vi "Practica 7 Case 2_0.vi"() -> ()   [LabVIEW 2020]
panel:
  out "VENTILADOR":bool
  out "LED":bool
  out "FOCO":bool
  out "Temp":dbl
  out "Ring":u16(ring)
  out "MENSAJE DE ADVERTENCIA":string
  in  "Sensor":dbl(slide) scale=0.0..50.0
  in  "TEMP MAX":dbl
  in  "TEMP MIN":dbl
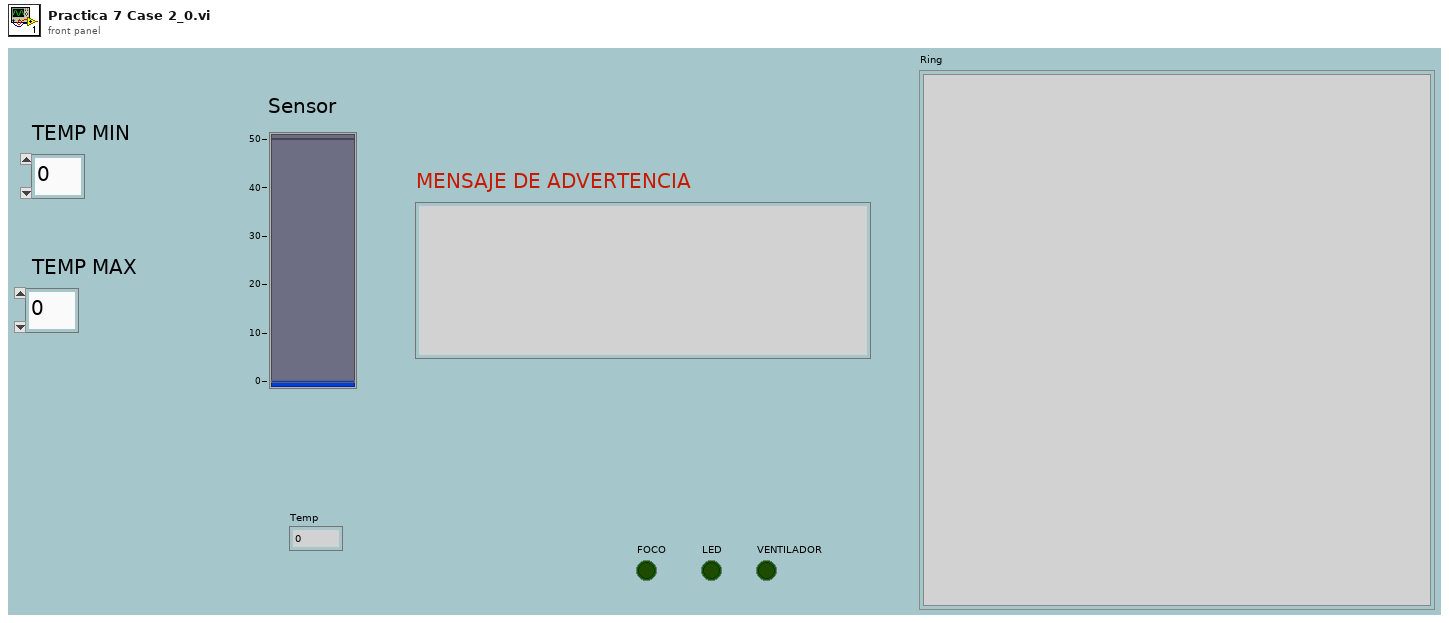
[diagram p1: front panel]
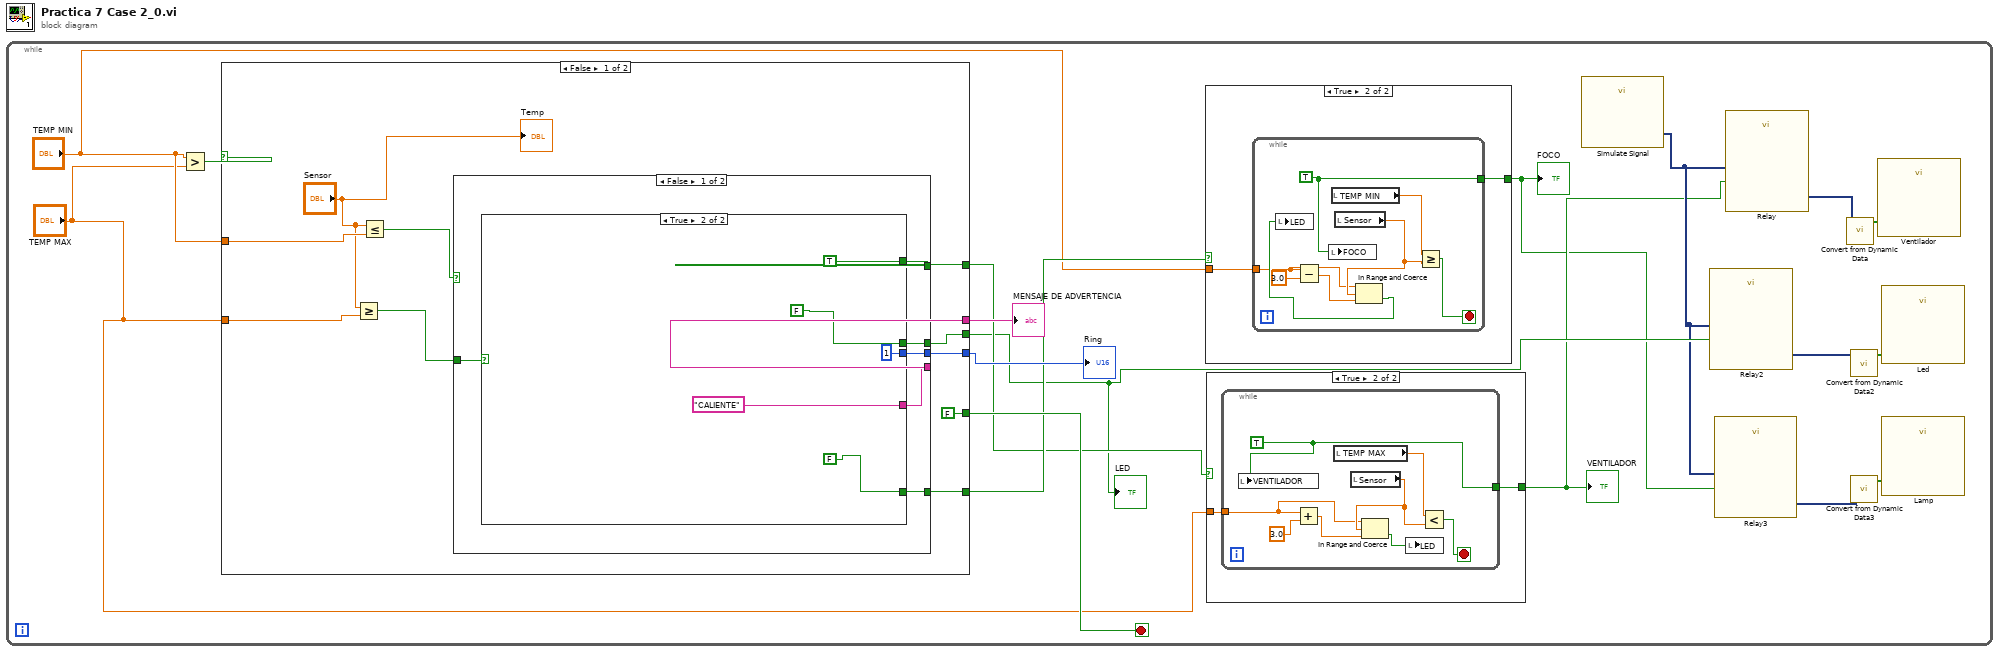
[diagram p0: block diagram]
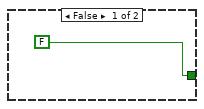
[diagram p2: hidden frame]
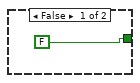
[diagram p3: hidden frame]
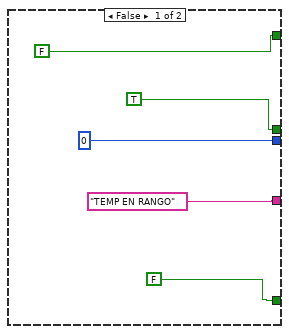
[diagram p4: hidden frame]
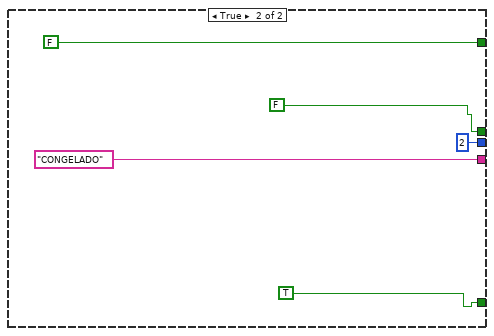
[diagram p5: hidden frame]
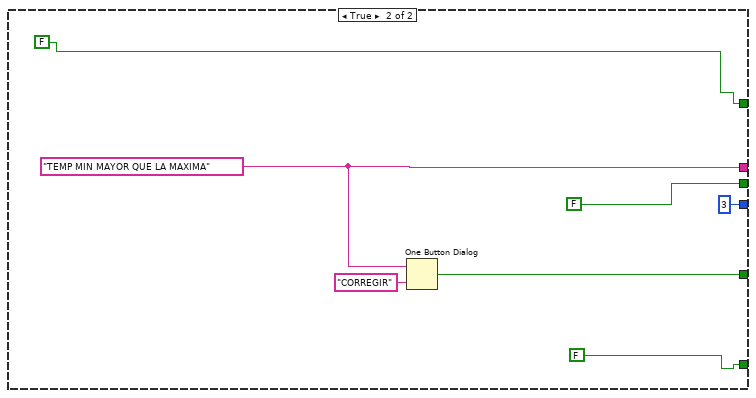
[diagram p6: hidden frame]
diagram:
  n1 = while {
    stop <- w15 stop-if-true
    n2 = Greater?(x="TEMP MIN", y="TEMP MAX") -> (0:w18:bool)
    n3 = case shown="False" w18 {
      tunnel: "TEMP MIN" -> [w50 _]
      tunnel: "TEMP MAX" -> [w51 _]
      tunnel: [w46 w77] -> w17
      tunnel: [w47 FALSE] -> w7
      tunnel: [w45 u16 3 ("Ring")] -> w16
      tunnel: [FALSE ("true") w76] -> w15
      tunnel: [w43 FALSE] -> w6
      tunnel: [w42 FALSE] -> w8
      frame False {
        n4 = Greater Or Equal?(x="Sensor", y=w51) -> (x >= y?=w48:bool)
        n5 = Less Or Equal?(x="Sensor", y=w50) -> (x <= y?=w49:bool)
        n6 = case shown="False" w49 {
          tunnel: w48 -> [w57 _]
          tunnel: [w56 FALSE] -> w47
          tunnel: [w55 "CONGELADO"] -> w46
          tunnel: [w54 u16 2 ("Ring")] -> w45
          tunnel: [w53 FALSE] -> w43
          tunnel: [w52 TRUE] -> w42
          frame False {
            n7 = case shown="True" w57 {
              tunnel: [FALSE TRUE] -> w56
              tunnel: ["TEMP EN RANGO" "CALIENTE"] -> w55
              tunnel: [u16 0 ("Ring") u16 1 ("Ring")] -> w54
              tunnel: [TRUE FALSE] -> w53
              tunnel: [FALSE FALSE] -> w52
              frame False {
              }
              frame True {
              }
            }
          }
          frame True {
          }
        }
        "Temp" <- "Sensor"
      }
      frame True {
        w77 = "TEMP MIN MAYOR QUE LA MAXIMA"
        n8 = One Button Dialog(message=w77, button name ("OK")="CORREGIR") -> (true=w76:bool)
      }
    }
    "MENSAJE DE ADVERTENCIA" <- w17
    "Ring" <- w16
    "LED" <- w6
    n9 = case shown="True" w8 {
      tunnel: [FALSE w32] -> w3
      tunnel: "TEMP MIN" -> [_ w31]
      frame False {
      }
      frame True {
        n10 = while {
          tunnel: [w39] -> w32
          tunnel: w31 -> [w33]
          stop <- w38 stop-if-true
          w39 = TRUE
          n11 = Subtract(x=w33, y=3.0) -> (x-y=w34:dbl)
          n12 = local write "FOCO"(w39) -> ()
          n13 = local read "TEMP MIN"() -> (w36:dbl)
          n14 = local read "Sensor"() -> (w35:dbl)
          n15 = In Range and Coerce(upper limit=w33, x=w35, lower limit=w34) -> (In Range?=w37:bool)  [unwired: 1 out]
          n16 = local write "LED"(w37) -> ()
          n17 = Greater Or Equal?(x=w36, y=w35) -> (x >= y?=w38:bool)
        }
      }
    }
    "FOCO" <- w3
    n18 = case shown="True" w7 {
      tunnel: [FALSE w21] -> w4
      tunnel: "TEMP MAX" -> [_ w20]
      frame False {
      }
      frame True {
        n19 = while {
          tunnel: [w28] -> w21
          tunnel: w20 -> [w22]
          stop <- w27 stop-if-true
          w28 = TRUE
          n20 = local write "VENTILADOR"(w28) -> ()
          n21 = Add(x=w22, y=3.0) -> (x+y=w23:dbl)
          n22 = local read "TEMP MAX"() -> (w25:dbl)
          n23 = local read "Sensor"() -> (w24:dbl)
          n24 = In Range and Coerce(upper limit=w22, x=w24, lower limit=w23) -> (In Range?=w26:bool)  [unwired: 1 out]
          n25 = local write "LED"(w26) -> ()
          n26 = Less?(x=w25, y=w24) -> (x < y?=w27:bool)
        }
      }
    }
    "VENTILADOR" <- w4
    n27 = call "Simulate Signal"() -> ("DC"=w5:dynamicdata)  [unwired: 14 in, 1 out]
    n28 = call "Relay2"("Enable"=w6, "Signals"=w5) -> ("Result"=w12:dynamicdata)  [unwired: 8 in, 1 out]
    n29 = call "Relay3"("Enable"=w3, "Signals"=w5) -> ("Result"=w10:dynamicdata)  [unwired: 8 in, 1 out]
    n30 = call "Relay"("Enable"=w4, "Signals"=w5) -> ("Result"=w14:dynamicdata)  [unwired: 8 in, 1 out]
    n31 = call "Convert from Dynamic Data"("Dynamic Data Type"=w14) -> ("Array"=w13:bool[])  [unwired: 3 in]
    n32 = call "Convert from Dynamic Data2"("Dynamic Data Type"=w12) -> ("Array"=w11:bool[])  [unwired: 3 in]
    n33 = call "Convert from Dynamic Data3"("Dynamic Data Type"=w10) -> ("Array"=w9:bool[])  [unwired: 3 in]
    n34 = call "Ventilador"("data"=w13) -> ()  [unwired: 17 in, 2 out]
    n35 = call "Led"("data"=w11) -> ()  [unwired: 17 in, 2 out]
    n36 = call "Lamp"("data"=w9) -> ()  [unwired: 17 in, 2 out]
  }
